vi "HFRR ADV v036.vi"() -> ()   [LabVIEW 2025] (continued)
            n1884 = local write "Main Dashboard Buttons"(T1."Advance" ("Main Dashboard Buttons")) -> ()
          }
        }
      }
    }
    n1885 = case shown="True" "Prog Uno" {
      frame False {
      }
      frame True {
        n1886 = stacked-sequence {
          frame #0 {
            n1887 = Delete(path (use dialog)=path "C:/LAB-IQ-NXT/UNOCOMPILE.bat" ("working directory")) -> ()  [unwired: 4 in, 3 out]
          }
          frame #1 {
            n1888 = local read "Com Port 1"() -> (w2646:refnum<visa-resource-name>)
            n1889 = Concatenate Strings("cmd.exe /c \"mode " ("command line"), w2646, ":1200,n,8,1\"\n" ("command line")) -> (w2651:string)
            n1890 = Concatenate Strings(w2651, "CD\\\nCD WinDucom\navrdude -C avrdude.conf -v -patmega328p -carduino -P" ("command line"), w2646, " -b115200 -D -Uflash:w:UNO_V20.hex:i\n" ("command line"), "\r") -> (w2653:string)
            "STR" <- w2653
            n1891 = call <vilib>:"Write Characters To File.vi"("append to file? (new file:F)"=FALSE, "character string"=w2653, "file path (dialog if empty)"=path "C:/LAB-IQ/UNOCOMPILE.bat" ("working directory")) -> ()  [unwired: 2 in, 1 out]
          }
          frame #2 {
            n1892 = disable-structure shown="Disabled" {
              frame Disabled {
                w2657 = "cmd.exe  /c \"C:\\LAB-IQ-NXT\\UNOCOMPILE.bat\"" ("string")
                n1893 = local write "Prog Uno"(FALSE ("run minimized? (F)")) -> ()
                n1894 = call <vilib>:"System Exec.vi"("expected output size  (4096)"=u32 65535, "run minimized? (F)"=FALSE, "wait until completion? (T)"=TRUE ("run minimized? (F)"), "working directory"=path "C:/LAB-IQ-NXT", "standard input"=w2657, "command line"=w2657) -> ("error out"=w2656:errorcluster, "standard output"=→"String 42":string)  [unwired: 2 in, 2 out]
                "error out 3" <- w2656
                n1895 = flat-sequence {
                  tunnel: w2656 -> [_]
                  frame #0 {
                  }
                }
              }
              frame Enabled {
              }
            }
          }
        }
      }
    }
    n1896 = case shown="\"ISO 12156\"" "TEST STANDARD" {
      frame "ASTM D6079", Default {
        w2626 = 50.0 ("Hz")
        w2627 = 53.0 ("Set Rh")
        w2629 = 1.0 ("Set Strk")
        w2628 = 60.0 ("Set Temp")
        # "astm hide"
        n1897 = local write "NORMAL LOAD"(200.0 ("NORMAL LOAD")) -> ()
        n1898 = local write "Set Strk"(w2629) -> ()
        n1899 = local write "Set Hz"(w2626) -> ()
        n1900 = local write "Set Temp"(w2628) -> ()
        n1901 = local write "Set Rh"(w2627) -> ()
        n1902 = local write "test time"(75.0 ("test time")) -> ()
        n1903 = local write "Set Stroke:"(w2629) -> ()
        n1904 = local write "Set Humidity:"(w2627) -> ()
        n1905 = local write "Set Frequency:"(w2626) -> ()
        n1906 = local write "Set Temperature:"(w2628) -> ()
        "Test Standard" <- "ASTM D6079" ("Test Standard 2")
      }
      frame "ISO 12156" {
        n1907 = local write "Set Strk"(1.0 ("Set Strk")) -> ()
        n1908 = local write "NORMAL LOAD"(200.0 ("NORMAL LOAD")) -> ()
        n1909 = local write "Set Temp"(60.0 ("Set Temp")) -> ()
        n1910 = local write "test time"(75.0 ("test time")) -> ()
        n1911 = local write "Set Hz"(50.0 ("Hz")) -> ()
        n1912 = local write "Set Rh"(53.0 ("Set Rh")) -> ()
      }
      frame "CEC F-096-A-06" {
        n1913 = local write "Set Strk"(1.0 ("Set Strk")) -> ()
        n1914 = local write "NORMAL LOAD"(200.0 ("NORMAL LOAD")) -> ()
        n1915 = local write "Set Temp"(60.0 ("Set Temp")) -> ()
        n1916 = local write "test time"(75.0 ("test time")) -> ()
        n1917 = local write "Set Hz"(50.0 ("Hz")) -> ()
        n1918 = local write "Set Rh"(53.0 ("Set Rh")) -> ()
      }
      frame "Custom" {
      }
    }
    n1919 = Or(x=w2179, y=w2177) -> (x .or. y?=w2178:bool)
    n1920 = case shown="\"About\"" w2176 {
      tunnel: [T29."Acquire" ("Main Tab") T29."Compare Files" ("Main Tab") T29."About" ("Main Tab")] -> w2187
      frame "Acquire", Default {
      }
      frame "Compare Files" {
      }
      frame "About" {
      }
    }
    n1921 = Or(x=w2182, y="OPEN") -> (x .or. y?=w2183:bool)
    n1922 = case shown="True" w2183 {
      tunnel: w2182 -> [_ w2215]
      frame False {
      }
      frame True {
        n1923 = stacked-sequence {
          tunnel: w2215 -> [_ w2282 _ _]
          frame #0 {
            w2231 = "  " ("String 6")
            n1924 = local write "OPEN"(FALSE ("open")) -> ()
            n1925 = local read "string1 2"() -> (w2219:string)
            n1926 = local read "string1 3"() -> (w2218:string)
            n1927 = local read "string1 4"() -> (w2217:string)
            n1928 = property on="OPEN" class="Bool (strict)"("Visible"=FALSE) -> ()  [unwired: 2 in, 2 out]
            n1929 = local write "String 6"(w2231) -> ()
            n1930 = local write "String 7"(w2231) -> ()
            n1931 = local write "String 8"(w2231) -> ()
            n1932 = local write "String 12"(w2231) -> ()
            n1933 = local read "OK Button 16"() -> (w2216:bool)
            n1934 = String To Path(string=w2219) -> (path=w2227:path)
            n1935 = String To Path(string=w2218) -> (path=w2226:path)
            n1936 = String To Path(string=w2217) -> (path=w2225:path)
            n1937 = case shown="True" w2216 {
              tunnel: [w2232 w2233] -> w2220
              frame False {
                n1938 = local read "string1"() -> (w2232:string)
              }
              frame True {
                n1939 = local read "String Indicator 4"() -> (w2233:string)
              }
            }
            n1940 = Open/Create/Replace File "Open File"(file path (use dialog)=w2227) -> (refnum out=w2223:refnum<file>)  [unwired: 5 in, 2 out]
            n1941 = Open/Create/Replace File "Open File"(file path (use dialog)=w2226) -> (refnum out=w2222:refnum<file>)  [unwired: 5 in, 2 out]
            n1942 = Open/Create/Replace File "Open File"(file path (use dialog)=w2225) -> (refnum out=w2221:refnum<file>)  [unwired: 5 in, 2 out]
            n1943 = while {
              tunnel: w2223 -> [w2245]
              i -> [w2241]
              stop <- w2240 continue-if-true
              (unwired) TRUE ("line mode (F)")
              n1944 = Read from Text File "Read File"(file (use dialog)=w2245) -> (text=w2242:string)  [unwired: 3 in, 3 out]
              n1945 = local write "Numeric 11"(w2241) -> ()
              n1946 = String Length(string=w2242) -> (length=w2244:i32)
              n1947 = Greater?(x=w2244, y=1) -> (0:w2240:bool)
            }
            n1948 = while {
              tunnel: w2222 -> [w2251]
              i -> [w2247]
              stop <- w2246 continue-if-true
              (unwired) TRUE ("line mode (F)")
              n1949 = Read from Text File "Read File"(file (use dialog)=w2251) -> (text=w2248:string)  [unwired: 3 in, 3 out]
              n1950 = local write "Numeric 12"(w2247) -> ()
              n1951 = String Length(string=w2248) -> (length=w2250:i32)
              n1952 = Greater?(x=w2250, y=1) -> (0:w2246:bool)
            }
            n1953 = while {
              tunnel: w2221 -> [w2257]
              i -> [w2253]
              stop <- w2252 continue-if-true
              (unwired) TRUE ("line mode (F)")
              n1954 = Read from Text File "Read File"(file (use dialog)=w2257) -> (text=w2254:string)  [unwired: 3 in, 3 out]
              n1955 = local write "Numeric 13"(w2253) -> ()
              n1956 = String Length(string=w2254) -> (length=w2256:i32)
              n1957 = Greater?(x=w2256, y=1) -> (0:w2252:bool)
            }
            n1958 = String To Path(string=w2220) -> (path=w2228:path)
            n1959 = Open/Create/Replace File "Open File"(file path (use dialog)=w2228) -> (refnum out=w2224:refnum<file>)  [unwired: 5 in, 2 out]
            n1960 = while {
              tunnel: w2224 -> [w2239]
              i -> [w2235]
              stop <- w2234 continue-if-true
              (unwired) TRUE ("line mode (F)")
              n1961 = Read from Text File "Read File"(file (use dialog)=w2239) -> (text=w2236:string)  [unwired: 3 in, 3 out]
              n1962 = local write "Numeric 8"(w2235) -> ()
              n1963 = String Length(string=w2236) -> (length=w2238:i32)
              n1964 = Greater?(x=w2238, y=1) -> (0:w2234:bool)
            }
          }
          frame #1 {
            w2409 = FALSE ("ACTUAL   MERGE")
            # "Sample Temp"
            # "ECR"
            # "COF"
            # "Time\nCOF\nFF\nTemp"
            n1965 = case shown="True" w2282 {
              tunnel: [w2429 w2430] -> w2283
              frame False {
                n1966 = local read "string1"() -> (w2429:string)
              }
              frame True {
                n1967 = local read "String Indicator 4"() -> (w2430:string)
              }
            }
            n1968 = local read "string1 3"() -> (w2327:string)
            n1969 = String To Path(string=w2283) -> (path=w2414:path)
            n1970 = String To Path(string=w2327) -> (path=w2425:path)
            n1971 = local read "Numeric 12"() -> (w2411:i32)
            n1972 = local read "Numeric 8"() -> (w2413:i32)
            n1973 = local read "string1 2"() -> (w2328:string)
            n1974 = local read "string1 4"() -> (w2326:string)
            n1975 = Open/Create/Replace File "Open File"(file path (use dialog)=w2414) -> (refnum out=w2428:refnum<file>, error out=w2427:errorcluster)  [unwired: 5 in, 1 out]
            n1976 = Open/Create/Replace File "Open File"(file path (use dialog)=w2425) -> (refnum out=w2421:refnum<file>, error out=w2422:errorcluster)  [unwired: 5 in, 1 out]
            n1977 = for {
              N: w2413 -> [_]
              tunnel: w2428 -> [w2576]
              tunnel: w2427 -> [w2575]
              tunnel: [w2565] -> w2340 mode=indexing
              tunnel: [w2563] -> w2397 mode=indexing
              tunnel: [w2564] -> w2392 mode=indexing
              tunnel: w2409 -> [_]
              tunnel: [w2557] -> w2394 mode=indexing
              tunnel: [w2553] -> w2363 mode=indexing
              tunnel: [w2549] -> w2338 mode=indexing
              tunnel: [w2545] -> w2319 mode=indexing
              tunnel: [w2540] -> w2279 mode=indexing
              (unwired) TRUE ("line mode (F)")
              # "freq"
              # "Stroke"
              # "Time"
              # "CoF"
              # "Humidity"
              # "Temp"
              # "Air Temp"
              # "ECR"
              n1978 = Read from Text File "Read File"(file (use dialog)=w2576, error in=w2575) -> (text=w2541:string)  [unwired: 2 in, 3 out]
              n1979 = local write "String 6"(w2541) -> ()
              n1980 = String Subset(string=w2541, offset (0)=0, length (rest)=14 ("length (rest)")) -> (substring=w2569:string)
              n1981 = String Subset(string=w2541, offset (0)=35, length (rest)=9 ("length (rest)")) -> (substring=w2566:string)
              n1982 = String Subset(string=w2541, offset (0)=15, length (rest)=9 ("length (rest)")) -> (substring=w2572:string)
              n1983 = Fract/Exp String To Number(string=w2569) -> (number=w2565:dbl)  [unwired: 3 in, 1 out]
              n1984 = Fract/Exp String To Number(string=w2566) -> (number=w2564:dbl)  [unwired: 3 in, 1 out]
              n1985 = Fract/Exp String To Number(string=w2572) -> (number=w2563:dbl)  [unwired: 3 in, 1 out]
              n1986 = String Subset(string=w2541, offset (0)=85, length (rest)=9 ("length (rest)")) -> (substring=w2542:string)
              n1987 = String Subset(string=w2541, offset (0)=25, length (rest)=9 ("length (rest)")) -> (substring=w2548:string)
              n1988 = String Subset(string=w2541, offset (0)=55, length (rest)=9 ("length (rest)")) -> (substring=w2550:string)
              n1989 = String Subset(string=w2541, offset (0)=45, length (rest)=9 ("length (rest)")) -> (substring=w2556:string)
              n1990 = String Subset(string=w2541, offset (0)=65, length (rest)=9 ("length (rest)")) -> (substring=w2562:string)
              n1991 = Fract/Exp String To Number(string=w2548) -> (number=w2545:dbl)  [unwired: 3 in, 1 out]
              n1992 = Fract/Exp String To Number(string=w2542) -> (number=w2540:dbl)  [unwired: 3 in, 1 out]
              n1993 = Fract/Exp String To Number(string=w2550) -> (number=w2549:dbl)  [unwired: 3 in, 1 out]
              n1994 = Fract/Exp String To Number(string=w2556) -> (number=w2553:dbl)  [unwired: 3 in, 1 out]
              n1995 = Fract/Exp String To Number(string=w2562) -> (number=w2559:dbl)  [unwired: 3 in, 1 out]
              n1996 = Add(x=w2559, y=0.0) -> (x+y=w2557:dbl)
            }
            n1997 = for {
              N: w2411 -> [_]
              tunnel: w2422 -> [w2502]
              tunnel: w2421 -> [w2501]
              tunnel: [w2491] -> w2380 mode=indexing
              tunnel: [w2489] -> w2378 mode=indexing
              tunnel: [w2490] -> w2374 mode=indexing
              tunnel: w2409 -> [_]
              tunnel: [w2483] -> w2376 mode=indexing
              tunnel: [w2479] -> w2358 mode=indexing
              tunnel: [w2475] -> w2334 mode=indexing
              tunnel: [w2472] -> w2315 mode=indexing
              tunnel: [w2468] -> w2274 mode=indexing
              (unwired) 9 ("length (rest)")
              (unwired) 9 ("length (rest)")
              (unwired) TRUE ("line mode (F)")
              n1998 = Read from Text File "Read File"(file (use dialog)=w2501, error in=w2502) -> (text=w2469:string)  [unwired: 2 in, 3 out]
              n1999 = local write "String 8"(w2469) -> ()
              n2000 = String Subset(string=w2469, offset (0)=85) -> (substring=w2471:string)  [unwired: 1 in]
              n2001 = String Subset(string=w2469, offset (0)=35, length (rest)=9 ("length (rest)")) -> (substring=w2492:string)
              n2002 = String Subset(string=w2469, offset (0)=55, length (rest)=9 ("length (rest)")) -> (substring=w2477:string)
              n2003 = String Subset(string=w2469, offset (0)=25) -> (substring=w2473:string)  [unwired: 1 in]
              n2004 = String Subset(string=w2469, offset (0)=15, length (rest)=9 ("length (rest)")) -> (substring=w2498:string)
              n2005 = String Subset(string=w2469, offset (0)=0, length (rest)=14 ("length (rest)")) -> (substring=w2495:string)
              n2006 = String Subset(string=w2469, offset (0)=45, length (rest)=9 ("length (rest)")) -> (substring=w2482:string)
              n2007 = String Subset(string=w2469, offset (0)=65, length (rest)=9 ("length (rest)")) -> (substring=w2488:string)
              n2008 = Fract/Exp String To Number(string=w2471) -> (number=w2468:dbl)  [unwired: 3 in, 1 out]
              n2009 = Fract/Exp String To Number(string=w2492) -> (number=w2490:dbl)  [unwired: 3 in, 1 out]
              n2010 = Fract/Exp String To Number(string=w2477) -> (number=w2475:dbl)  [unwired: 3 in, 1 out]
              n2011 = Fract/Exp String To Number(string=w2473) -> (number=w2472:dbl)  [unwired: 3 in, 1 out]
              n2012 = Fract/Exp String To Number(string=w2498) -> (number=w2489:dbl)  [unwired: 3 in, 1 out]
              n2013 = Fract/Exp String To Number(string=w2495) -> (number=w2491:dbl)  [unwired: 3 in, 1 out]
              n2014 = Fract/Exp String To Number(string=w2482) -> (number=w2479:dbl)  [unwired: 3 in, 1 out]
              n2015 = Fract/Exp String To Number(string=w2488) -> (number=w2485:dbl)  [unwired: 3 in, 1 out]
              n2016 = Add(x=w2485, y=0.0) -> (x+y=w2483:dbl)
            }
            n2017 = String To Path(string=w2328) -> (path=w2426:path)
            n2018 = String To Path(string=w2326) -> (path=w2420:path)
            n2019 = local read "Numeric 11"() -> (w2410:i32)
            n2020 = local read "Numeric 13"() -> (w2412:i32)
            n2021 = Open/Create/Replace File "Open File"(file path (use dialog)=w2426) -> (refnum out=w2424:refnum<file>, error out=w2423:errorcluster)  [unwired: 5 in, 1 out]
            n2022 = Open/Create/Replace File "Open File"(file path (use dialog)=w2420) -> (refnum out=w2419:refnum<file>, error out=w2418:errorcluster)  [unwired: 5 in, 1 out]
            n2023 = for {
              N: w2410 -> [_]
              tunnel: w2424 -> [w2539]
              tunnel: w2423 -> [w2538]
              tunnel: [w2528] -> w2390 mode=indexing
              tunnel: [w2526] -> w2388 mode=indexing
              tunnel: [w2527] -> w2383 mode=indexing
              tunnel: w2409 -> [_]
              tunnel: [w2520] -> w2385 mode=indexing
              tunnel: [w2516] -> w2361 mode=indexing
              tunnel: [w2512] -> w2336 mode=indexing
              tunnel: [w2508] -> w2317 mode=indexing
              tunnel: [w2503] -> w2275 mode=indexing
              (unwired) TRUE ("line mode (F)")
              n2024 = Read from Text File "Read File"(file (use dialog)=w2539, error in=w2538) -> (text=w2504:string)  [unwired: 2 in, 3 out]
              n2025 = local write "String 7"(w2504) -> ()
              n2026 = String Subset(string=w2504, offset (0)=85, length (rest)=9 ("length (rest)")) -> (substring=w2507:string)
              n2027 = String Subset(string=w2504, offset (0)=35, length (rest)=9 ("length (rest)")) -> (substring=w2529:string)
              n2028 = String Subset(string=w2504, offset (0)=55, length (rest)=9 ("length (rest)")) -> (substring=w2515:string)
              n2029 = String Subset(string=w2504, offset (0)=25, length (rest)=9 ("length (rest)")) -> (substring=w2509:string)
              n2030 = String Subset(string=w2504, offset (0)=45, length (rest)=9 ("length (rest)")) -> (substring=w2517:string)
              n2031 = String Subset(string=w2504, offset (0)=0, length (rest)=14 ("length (rest)")) -> (substring=w2532:string)
              n2032 = String Subset(string=w2504, offset (0)=15, length (rest)=9 ("length (rest)")) -> (substring=w2535:string)
              n2033 = String Subset(string=w2504, offset (0)=65, length (rest)=9 ("length (rest)")) -> (substring=w2521:string)
              n2034 = Fract/Exp String To Number(string=w2507) -> (number=w2503:dbl)  [unwired: 3 in, 1 out]
              n2035 = Fract/Exp String To Number(string=w2529) -> (number=w2527:dbl)  [unwired: 3 in, 1 out]
              n2036 = Fract/Exp String To Number(string=w2515) -> (number=w2512:dbl)  [unwired: 3 in, 1 out]
              n2037 = Fract/Exp String To Number(string=w2509) -> (number=w2508:dbl)  [unwired: 3 in, 1 out]
              n2038 = Fract/Exp String To Number(string=w2517) -> (number=w2516:dbl)  [unwired: 3 in, 1 out]
              n2039 = Fract/Exp String To Number(string=w2532) -> (number=w2528:dbl)  [unwired: 3 in, 1 out]
              n2040 = Fract/Exp String To Number(string=w2535) -> (number=w2526:dbl)  [unwired: 3 in, 1 out]
              n2041 = Fract/Exp String To Number(string=w2521) -> (number=w2524:dbl)  [unwired: 3 in, 1 out]
              n2042 = Add(x=w2524, y=0.0) -> (x+y=w2520:dbl)
            }
            n2043 = for {
              N: w2412 -> [_]
              tunnel: w2419 -> [w2467]
              tunnel: w2418 -> [w2466]
              tunnel: [w2456] -> w2372 mode=indexing
              tunnel: [w2455] -> w2365 mode=indexing
              tunnel: w2409 -> [_]
              tunnel: [w2444] -> w2370 mode=indexing
              tunnel: [w2449] -> w2367 mode=indexing
              tunnel: [w2445] -> w2357 mode=indexing
              tunnel: [w2440] -> w2332 mode=indexing
              tunnel: [w2436] -> w2313 mode=indexing
              tunnel: [w2431] -> w2273 mode=indexing
              (unwired) 1.0 ("x")
              (unwired) TRUE ("line mode (F)")
              n2044 = Read from Text File "Read File"(file (use dialog)=w2467, error in=w2466) -> (text=w2432:string)  [unwired: 2 in, 3 out]
              n2045 = local write "String 12"(w2432) -> ()
              n2046 = String Subset(string=w2432, offset (0)=85, length (rest)=9 ("length (rest)")) -> (substring=w2434:string)
              n2047 = String Subset(string=w2432, offset (0)=35, length (rest)=9 ("length (rest)")) -> (substring=w2457:string)
              n2048 = String Subset(string=w2432, offset (0)=55, length (rest)=9 ("length (rest)")) -> (substring=w2442:string)
              n2049 = String Subset(string=w2432, offset (0)=25, length (rest)=9 ("length (rest)")) -> (substring=w2438:string)
              n2050 = String Subset(string=w2432, offset (0)=45, length (rest)=9 ("length (rest)")) -> (substring=w2447:string)
              n2051 = String Subset(string=w2432, offset (0)=15, length (rest)=9 ("length (rest)")) -> (substring=w2463:string)
              n2052 = String Subset(string=w2432, offset (0)=0, length (rest)=14 ("length (rest)")) -> (substring=w2460:string)
              n2053 = String Subset(string=w2432, offset (0)=65, length (rest)=9 ("length (rest)")) -> (substring=w2450:string)
              n2054 = Fract/Exp String To Number(string=w2434) -> (number=w2431:dbl)  [unwired: 3 in, 1 out]
              n2055 = Fract/Exp String To Number(string=w2457) -> (number=w2455:dbl)  [unwired: 3 in, 1 out]
              n2056 = Fract/Exp String To Number(string=w2442) -> (number=w2440:dbl)  [unwired: 3 in, 1 out]
              n2057 = Fract/Exp String To Number(string=w2438) -> (number=w2436:dbl)  [unwired: 3 in, 1 out]
              n2058 = Fract/Exp String To Number(string=w2447) -> (number=w2445:dbl)  [unwired: 3 in, 1 out]
              n2059 = Fract/Exp String To Number(string=w2463) -> (number=w2444:dbl)  [unwired: 3 in, 1 out]
              n2060 = Fract/Exp String To Number(string=w2460) -> (number=w2456:dbl)  [unwired: 3 in, 1 out]
              n2061 = Fract/Exp String To Number(string=w2450) -> (number=w2453:dbl)  [unwired: 3 in, 1 out]
              n2062 = Add(x=w2453, y=0.0) -> (x+y=w2449:dbl)
            }
            n2063 = Delete From Array(array=w2315, index=0) -> (array with subset deleted=w2288:dbl[])  [unwired: 1 in, 1 out]
            n2064 = Delete From Array(array=w2378, index=0) -> (array with subset deleted=w2351:dbl[])  [unwired: 1 in, 1 out]
            n2065 = Delete From Array(array=w2358, index=0) -> (array with subset deleted=w2346:dbl[])  [unwired: 1 in, 1 out]
            n2066 = Delete From Array(array=w2376, index=0) -> (array with subset deleted=w2377:dbl[])  [unwired: 1 in, 1 out]
            n2067 = call-poly <vilib>:"Mean.vi"("X"=w2288) -> ("mean"=→"КОФ2 4":dbl)  [unwired: 1 out]
            n2068 = call-poly <vilib>:"Mean.vi"("X"=w2351) -> ("mean"=→"КОФ3":dbl)  [unwired: 1 out]
            n2069 = call-poly <vilib>:"Mean.vi"("X"=w2346) -> ("mean"=→"CP3":dbl)  [unwired: 1 out]
            n2070 = Delete From Array(array=w2340, index=0) -> (array with subset deleted=w2267:dbl[])  [unwired: 1 in, 1 out]
            n2071 = Delete From Array(array=w2279, index=0) -> (array with subset deleted=w2266:dbl[])  [unwired: 1 in, 1 out]
            n2072 = Delete From Array(array=w2319, index=0) -> (array with subset deleted=w2290:dbl[])  [unwired: 1 in, 1 out]
            n2073 = Delete From Array(array=w2397, index=0) -> (array with subset deleted=w2352:dbl[])  [unwired: 1 in, 1 out]
            n2074 = Delete From Array(array=w2363, index=0) -> (array with subset deleted=w2348:dbl[])  [unwired: 1 in, 1 out]
            "array w/ subset deleted" <- w2348
            n2075 = Delete From Array(array=w2394, index=0) -> (array with subset deleted=w2395:dbl[])  [unwired: 1 in, 1 out]
            n2076 = call-poly <vilib>:"Mean.vi"("X"=w2290) -> ("mean"=→"КОФ2 2":dbl)  [unwired: 1 out]
            n2077 = call-poly <vilib>:"Mean.vi"("X"=w2352) -> ("mean"=→"КОФ1":dbl)  [unwired: 1 out]
            n2078 = Bundle "Bundle"(w2267, w2266) -> (w2272:cluster{dbl[], dbl[]})  [unwired: 1 in]
            n2079 = Bundle "Bundle"(w2267, w2395) -> (w2259:cluster{dbl[], dbl[]})  [unwired: 1 in]
            n2080 = Delete From Array(array=w2274, index=0) -> (array with subset deleted=w2262:dbl[])  [unwired: 1 in, 1 out]
            n2081 = Delete From Array(array=w2275, index=0) -> (array with subset deleted=w2264:dbl[])  [unwired: 1 in, 1 out]
            n2082 = Delete From Array(array=w2385, index=0) -> (array with subset deleted=w2386:dbl[])  [unwired: 1 in, 1 out]
            n2083 = Delete From Array(array=w2273, index=0) -> (array with subset deleted=w2260:dbl[])  [unwired: 1 in, 1 out]
            n2084 = Delete From Array(array=w2367, index=0) -> (array with subset deleted=w2368:dbl[])  [unwired: 1 in, 1 out]
            n2085 = Delete From Array(array=w2392, index=0) -> (array with subset deleted=w2298:dbl[])  [unwired: 1 in, 1 out]
            n2086 = Delete From Array(array=w2338, index=0) -> (array with subset deleted=w2294:dbl[])  [unwired: 1 in, 1 out]
            n2087 = Delete From Array(array=w2374, index=0) -> (array with subset deleted=w2296:dbl[])  [unwired: 1 in, 1 out]
            n2088 = Delete From Array(array=w2334, index=0) -> (array with subset deleted=w2292:dbl[])  [unwired: 1 in, 1 out]
            n2089 = Delete From Array(array=w2383, index=0) -> (array with subset deleted=w2297:dbl[])  [unwired: 1 in, 1 out]
            n2090 = Delete From Array(array=w2336, index=0) -> (array with subset deleted=w2293:dbl[])  [unwired: 1 in, 1 out]
            n2091 = Delete From Array(array=w2317, index=0) -> (array with subset deleted=w2289:dbl[])  [unwired: 1 in, 1 out]
            n2092 = Delete From Array(array=w2361, index=0) -> (array with subset deleted=w2347:dbl[])  [unwired: 1 in, 1 out]
            n2093 = Delete From Array(array=w2388, index=0) -> (array with subset deleted=w2349:dbl[])  [unwired: 1 in, 1 out]
            n2094 = Delete From Array(array=w2365, index=0) -> (array with subset deleted=w2295:dbl[])  [unwired: 1 in, 1 out]
            n2095 = Delete From Array(array=w2332, index=0) -> (array with subset deleted=w2291:dbl[])  [unwired: 1 in, 1 out]
            n2096 = Delete From Array(array=w2313, index=0) -> (array with subset deleted=w2287:dbl[])  [unwired: 1 in, 1 out]
            n2097 = Delete From Array(array=w2357, index=0) -> (array with subset deleted=w2345:dbl[])  [unwired: 1 in, 1 out]
            n2098 = Delete From Array(array=w2370, index=0) -> (array with subset deleted=w2350:dbl[])  [unwired: 1 in, 1 out]
            n2099 = Delete From Array(array=w2380, index=0) -> (array with subset deleted=w2263:dbl[])  [unwired: 1 in, 1 out]
            n2100 = Delete From Array(array=w2390, index=0) -> (array with subset deleted=w2265:dbl[])  [unwired: 1 in, 1 out]
            n2101 = Delete From Array(array=w2372, index=0) -> (array with subset deleted=w2261:dbl[])  [unwired: 1 in, 1 out]
            n2102 = Bundle "Bundle"(w2267, w2298) -> (w2285:cluster{dbl[], dbl[]})  [unwired: 1 in]
            n2103 = Bundle "Bundle"(w2267, w2352) -> (w2286:cluster{dbl[], dbl[]})  [unwired: 1 in]
            n2104 = Bundle "Bundle"(w2298, w2294) -> (w2300:cluster{dbl[], dbl[]})  [unwired: 1 in]
            n2105 = Bundle "Bundle"(w2263, w2262) -> (w2270:cluster{dbl[], dbl[]})  [unwired: 1 in]
            n2106 = Bundle "Bundle"(w2296, w2292) -> (w2302:cluster{dbl[], dbl[]})  [unwired: 1 in]
            n2107 = Bundle "Bundle"(w2263, w2296) -> (w2406:cluster{dbl[], dbl[]})  [unwired: 1 in]
            n2108 = Bundle "Bundle"(w2263, w2292) -> (w2330:cluster{dbl[], dbl[]})  [unwired: 1 in]
            n2109 = Bundle "Bundle"(w2263, w2351) -> (w2416:cluster{dbl[], dbl[]})  [unwired: 1 in]
            n2110 = Bundle "Bundle"(w2263, w2346) -> (w2354:cluster{dbl[], dbl[]})  [unwired: 1 in]
            n2111 = Bundle "Bundle"(w2263, w2377) -> (w2401:cluster{dbl[], dbl[]})  [unwired: 1 in]
            n2112 = Bundle "Bundle"(w2297, w2293) -> (w2301:cluster{dbl[], dbl[]})  [unwired: 1 in]
            n2113 = Bundle "Bundle"(w2265, w2264) -> (w2271:cluster{dbl[], dbl[]})  [unwired: 1 in]
            n2114 = Bundle "Bundle"(w2265, w2297) -> (w2408:cluster{dbl[], dbl[]})  [unwired: 1 in]
            n2115 = Bundle "Bundle"(w2265, w2293) -> (w2331:cluster{dbl[], dbl[]})  [unwired: 1 in]
            n2116 = Bundle "Bundle"(w2265, w2347) -> (w2355:cluster{dbl[], dbl[]})  [unwired: 1 in]
            n2117 = Bundle "Bundle"(w2265, w2349) -> (w2417:cluster{dbl[], dbl[]})  [unwired: 1 in]
            n2118 = Bundle "Bundle"(w2265, w2386) -> (w2399:cluster{dbl[], dbl[]})  [unwired: 1 in]
            n2119 = Bundle "Bundle"(w2295, w2291) -> (w2303:cluster{dbl[], dbl[]})  [unwired: 1 in]
            n2120 = Bundle "Bundle"(w2261, w2260) -> (w2269:cluster{dbl[], dbl[]})  [unwired: 1 in]
            n2121 = Bundle "Bundle"(w2261, w2295) -> (w2407:cluster{dbl[], dbl[]})  [unwired: 1 in]
            n2122 = Bundle "Bundle"(w2261, w2291) -> (w2329:cluster{dbl[], dbl[]})  [unwired: 1 in]
            n2123 = Bundle "Bundle"(w2261, w2345) -> (w2353:cluster{dbl[], dbl[]})  [unwired: 1 in]
            n2124 = Bundle "Bundle"(w2261, w2350) -> (w2415:cluster{dbl[], dbl[]})  [unwired: 1 in]
            n2125 = Bundle "Bundle"(w2261, w2368) -> (w2400:cluster{dbl[], dbl[]})  [unwired: 1 in]
            n2126 = call-poly <vilib>:"Mean.vi"("X"=w2348) -> ("mean"=→"CP1":dbl)  [unwired: 1 out]
            n2127 = call-poly <vilib>:"Mean.vi"("X"=w2289) -> ("mean"=→"КОФ2 3":dbl)  [unwired: 1 out]
            n2128 = call-poly <vilib>:"Mean.vi"("X"=w2347) -> ("mean"=→"CP2":dbl)  [unwired: 1 out]
            n2129 = call-poly <vilib>:"Mean.vi"("X"=w2349) -> ("mean"=→"КОФ2":dbl)  [unwired: 1 out]
            n2130 = call-poly <vilib>:"Mean.vi"("X"=w2287) -> ("mean"=→"КОФ2 5":dbl)  [unwired: 1 out]
            n2131 = call-poly <vilib>:"Mean.vi"("X"=w2345) -> ("mean"=→"CP4":dbl)  [unwired: 1 out]
            n2132 = call-poly <vilib>:"Mean.vi"("X"=w2350) -> ("mean"=→"КОФ4":dbl)  [unwired: 1 out]
            n2133 = Bundle "Bundle"(w2267, w2294) -> (w2258:cluster{dbl[], dbl[]})  [unwired: 1 in]
            n2134 = Bundle "Bundle"(w2267, w2348) -> (w2281:cluster{dbl[], dbl[]})  [unwired: 1 in]
            n2135 = Build Array "Build Array"(w2258, w2281) -> (w2284:cluster{dbl[], dbl[]}[])
            "XY Graph 17" <- w2284
            n2136 = Build Array "Build Array"(w2272, w2271, w2270, w2269) -> (→"Frequency ( Hz )":cluster{dbl[], dbl[]}[])
            n2137 = Build Array "Build Array"(w2300, w2301, w2302, w2303) -> (→"Air Temp ( °C ) vs Humidity ( % RH )":cluster{dbl[], dbl[]}[])
            n2138 = Build Array "Build Array"(w2285, w2408, w2406, w2407) -> (→"Air Temperature  ( °C )":cluster{dbl[], dbl[]}[])
            n2139 = Build Array "Build Array"(w2258, w2331, w2330, w2329) -> (→"Humidity ( %RH )":cluster{dbl[], dbl[]}[])
            n2140 = Build Array "Build Array"(w2286, w2417, w2416, w2415) -> (→"Coefficient Of Friction":cluster{dbl[], dbl[]}[])
            n2141 = Build Array "Build Array"(w2281, w2355, w2354, w2353) -> (→"Sample Temperature ( °C )":cluster{dbl[], dbl[]}[])
            n2142 = Build Array "Build Array"(w2259, w2399, w2401, w2400) -> (→"XY Graph 13":cluster{dbl[], dbl[]}[])
            n2143 = Bundle "Bundle"(w2267, w2290) -> (w2312:cluster{dbl[], dbl[]})  [unwired: 1 in]
            n2144 = Bundle "Bundle"(w2263, w2288) -> (w2310:cluster{dbl[], dbl[]})  [unwired: 1 in]
            n2145 = Bundle "Bundle"(w2265, w2289) -> (w2311:cluster{dbl[], dbl[]})  [unwired: 1 in]
            n2146 = Bundle "Bundle"(w2261, w2287) -> (w2309:cluster{dbl[], dbl[]})  [unwired: 1 in]
            n2147 = Build Array "Build Array"(w2312, w2311, w2310, w2309) -> (→"Stroke ( mm )":cluster{dbl[], dbl[]}[])
            n2148 = local write "XY Graph 16"(w2284) -> ()
          }
          frame #2 {
          }
          frame #3 {
            n2149 = local write "Numeric 8"(0 ("Numeric 8")) -> ()
            n2150 = local write "Numeric 11"(0 ("Numeric 11")) -> ()
            n2151 = local write "Numeric 12"(0 ("Numeric 12")) -> ()
            n2152 = local write "Numeric 13"(0 ("Numeric 13")) -> ()
            n2153 = property on="OPEN" class="Bool (strict)"("Visible"=TRUE) -> ()  [unwired: 2 in, 2 out]
            n2154 = local read "String Control 2"() -> (w2584:string)
            n2155 = local read "String Control 4"() -> (w2583:string)
            n2156 = local read "String Control 6"() -> (w2582:string)
            n2157 = local read "String Control 8"() -> (w2581:string)
            n2158 = Match Pattern(string=w2584, regular expression="Samples / cycle :- ") -> (after substring=w2598:string)  [unwired: 1 in, 3 out]
            n2159 = Match Pattern(string=w2584, regular expression="Frequency :- ") -> (after substring=w2617:string)  [unwired: 1 in, 3 out]
            n2160 = Match Pattern(string=w2583, regular expression="Samples / cycle :- ") -> (after substring=w2594:string)  [unwired: 1 in, 3 out]
            n2161 = Match Pattern(string=w2583, regular expression="Frequency :- ") -> (after substring=w2612:string)  [unwired: 1 in, 3 out]
            n2162 = Match Pattern(string=w2582, regular expression="Samples / cycle :- ") -> (after substring=w2590:string)  [unwired: 1 in, 3 out]
            n2163 = Match Pattern(string=w2582, regular expression="Frequency :- ") -> (after substring=w2607:string)  [unwired: 1 in, 3 out]
            n2164 = Match Pattern(string=w2581, regular expression="Samples / cycle :- ") -> (after substring=w2586:string)  [unwired: 1 in, 3 out]
            n2165 = Match Pattern(string=w2581, regular expression="Frequency :- ") -> (after substring=w2602:string)  [unwired: 1 in, 3 out]
            n2166 = String Subset(string=w2598, length (rest)=6 ("length (rest)")) -> (substring=w2600:string)  [unwired: 1 in]
            n2167 = String Subset(string=w2617, length (rest)=9 ("length (rest)")) -> (substring=w2619:string)  [unwired: 1 in]
            n2168 = String Subset(string=w2594, length (rest)=6 ("length (rest)")) -> (substring=w2596:string)  [unwired: 1 in]
            n2169 = String Subset(string=w2612, length (rest)=9 ("length (rest)")) -> (substring=w2614:string)  [unwired: 1 in]
            n2170 = String Subset(string=w2590, length (rest)=6 ("length (rest)")) -> (substring=w2592:string)  [unwired: 1 in]
            n2171 = String Subset(string=w2607, length (rest)=9 ("length (rest)")) -> (substring=w2609:string)  [unwired: 1 in]
            n2172 = String Subset(string=w2586, length (rest)=6 ("length (rest)")) -> (substring=w2588:string)  [unwired: 1 in]
            n2173 = String Subset(string=w2602, length (rest)=9 ("length (rest)")) -> (substring=w2604:string)  [unwired: 1 in]
            n2174 = Fract/Exp String To Number(string=w2600) -> (number=w2580:dbl)  [unwired: 3 in, 1 out]
            n2175 = Fract/Exp String To Number(string=w2619) -> (number=w2620:dbl)  [unwired: 3 in, 1 out]
            n2176 = Fract/Exp String To Number(string=w2596) -> (number=w2579:dbl)  [unwired: 3 in, 1 out]
            n2177 = Fract/Exp String To Number(string=w2614) -> (number=w2615:dbl)  [unwired: 3 in, 1 out]
            n2178 = Fract/Exp String To Number(string=w2592) -> (number=w2578:dbl)  [unwired: 3 in, 1 out]
            n2179 = Fract/Exp String To Number(string=w2609) -> (number=w2610:dbl)  [unwired: 3 in, 1 out]
            n2180 = Fract/Exp String To Number(string=w2588) -> (number=w2577:dbl)  [unwired: 3 in, 1 out]
            n2181 = Fract/Exp String To Number(string=w2604) -> (number=w2605:dbl)  [unwired: 3 in, 1 out]
            n2182 = local write "sample1"(w2580) -> ()
            n2183 = local write "freq1"(w2620) -> ()
            n2184 = local write "sample2"(w2579) -> ()
            n2185 = local write "freq2"(w2615) -> ()
            n2186 = local write "sample3"(w2578) -> ()
            n2187 = local write "freq3"(w2610) -> ()
            n2188 = local write "sample4"(w2577) -> ()
            n2189 = local write "freq 4"(w2605) -> ()
          }
        }
      }
    }
    n2190 = case shown="True" w2178 {
      selector: w2178 -> [_ w2197]
      frame False {
      }
      frame True {
        n2191 = Not(x=w2197) -> (.not. x?=w2193:bool)
        n2192 = local write "service 3"(w2193) -> ()
        n2193 = local write "OPEN 6"(w2193) -> ()
        n2194 = call <vilib>:"System Exec.vi"("wait until completion? (T)"=TRUE, "command line"="C:\\LAB-IQ\\Scar View.exe") -> ("error out"=→"error out 5":errorcluster)  [unwired: 6 in, 3 out]
      }
    }
    n2195 = case shown="\"Acquire\", Default" w2187 {
      frame "Acquire", Default {
        # "Elapsed time\ncof\nstroke\nAir temp\nTemp\nHumidity"
        n2196 = disable-structure shown="Disabled" {
          frame Disabled {
            n2197 = local read "Flag"() -> (w2896:dbl)
            n2198 = local read "RUN"() -> (w2893:bool)
            n2199 = Not(x=w2893) -> (.not. x?=w2892:bool)
            n2200 = Equal?(x=w2896, y=10.0) -> (x = y?=w2894:bool)
            n2201 = And(x=w2894, y=w2892) -> (x .and. y?=w2891:bool)
            n2202 = case shown="True" w2891 {
              frame False {
              }
              frame True {
                w2897 = FALSE ("Heater Button")
                n2203 = local write "Humidity"(w2897) -> ()
                n2204 = local write "Heater Button"(w2897) -> ()
              }
            }
          }
          frame Enabled {
          }
        }
        n2205 = disable-structure shown="Disabled" {
          frame Disabled {
            n2206 = case shown="True" {
              selector: _ -> [_ _]
              frame False {
              }
              frame True {
                w2942 = TRUE ("Heater")
                n2207 = local write "Humidity"(w2942) -> ()
                n2208 = local write "Heater Button"(w2942) -> ()
                n2209 = local read "TEST STANDARD"() -> (w2945:T3)
                n2210 = local read "TEST STANDARD"() -> (w2940:T3)
                n2211 = Equal?(x=w2945, y=enum16{"ASTM D6079", "ISO 12156", "Custom"}."ISO 12156" ("Test Standard")) -> (x = y?=w2943:bool)
                n2212 = Equal?(x=w2940, y=enum16{"ASTM D6079", "ISO 12156", "Custom"}."ASTM D6079" ("Test Standard")) -> (x = y?=w2939:bool)
                n2213 = case shown="True" w2943 {
                  frame False {
                  }
                  frame True {
                    n2214 = local write "airtempflg"(FALSE ("airtempflg")) -> ()
                    n2215 = local write item#-1(TRUE ("Heater")) -> ()
                  }
                }
                n2216 = case shown="True" w2939 {
                  frame False {
                  }
                  frame True {
                    n2217 = local write "airtempflg"(TRUE ("airtempflg")) -> ()
                    n2218 = local write item#-1(FALSE ("Heater")) -> ()
                  }
                }
              }
            }
          }
          frame Enabled {
          }
        }
        n2219 = stacked-sequence {
          frame #0 {
            n2220 = case shown="True" "RST FF" {
              frame False {
              }
              frame True {
                w2959 = 0.0 ("X Scale.Range:Maximum")
                n2221 = property on="Frictional Force ( N )" class="WFChart (strict)"("XScale.Maximum"=600.0 ("X Scale.Range:Maximum"), "XScale.Minimum"=w2959, "YScale.Maximum"=10.0 ("Y Scale.Range:Maximum"), "YScale.Minimum"=w2959) -> ()  [unwired: 2 in, 2 out]
              }
            }
          }
          frame #1 {
            n2222 = case shown="True" "RST TEMP" {
              frame False {
              }
              frame True {
                n2223 = property on="Temperature ( Deg C )" class="WFChart (strict)"("XScale.Minimum"=0.0 ("X Scale.Range:Minimum"), "XScale.Maximum"=600.0 ("X Scale.Range:Maximum"), "YScale.Minimum"=0.0 ("Y Scale.Range:Minimum"), "YScale.Maximum"=100.0 ("Y Scale.Range:Maximum")) -> ()  [unwired: 2 in, 2 out]
              }
            }
          }
          frame #2 {
            n2224 = case shown="True" "RSTCOF" {
              frame False {
              }
              frame True {
                n2225 = property on="Coefficient of Friction" class="WFChart (strict)"("XScale.Minimum"=0.0 ("X Scale.Range:Minimum"), "XScale.Maximum"=600.0 ("X Scale.Range:Maximum"), "YScale.Maximum"=1.0 ("X Scale.Range:Minimum"), "YScale.Minimum"=0.0 ("X Scale.Range:Minimum")) -> ()  [unwired: 2 in, 2 out]
              }
            }
          }
          frame #3 {
            n2226 = case shown="True" "RSTCOF 2" {
              frame False {
              }
              frame True {
                (unwired) 100.0 ("Y Scale.Range:Maximum")
                (unwired) 0.0 ("Y Scale.Range:Minimum")
                (unwired) 600.0 ("X Scale.Range:Maximum")
                (unwired) 0.0 ("X Scale.Range:Minimum")
              }
            }
          }
          frame #4 {
            n2227 = case shown="True" "RSTCOF 3" {
              frame False {
              }
              frame True {
                n2228 = property on="Electrical Contact Resistance ( % )" class="WFChart (strict)"("XScale.Minimum"=0.0 ("X Scale.Range:Minimum"), "XScale.Maximum"=600.0 ("X Scale.Range:Maximum"), "YScale.Minimum"=0.0 ("Y Scale.Range:Minimum"), "YScale.Maximum"=100.0 ("Y Scale.Range:Maximum")) -> ()  [unwired: 2 in, 2 out]
              }
            }
          }
        }
        n2229 = local read "RUN"() -> (w2886:bool)
        n2230 = case shown="False" w2886 {
          frame False {
          }
          frame True {
          }
        }
        n2231 = local read "RUN"() -> (w2890:bool)
        n2232 = case shown="False" w2890 {
          tunnel: [FALSE ("TEST RUNNING") TRUE ("TEST RUNNING")] -> w2889
          frame False {
            w2978 = 0.0 ("Flag")
            n2233 = local write "Elapsed time"(0.0 ("elapsedtime")) -> ()
            n2234 = local write "Time Remaining"(w2978) -> ()
            n2235 = local write "Flag"(w2978) -> ()
            n2236 = local write "Remaining Time"(w2978) -> ()
          }
          frame True {
            n2237 = local write "Flag"(10.0 ("Flag")) -> ()
          }
        }
        n2238 = local read "AIR TEMP"() -> (w2884:dbl)
        n2239 = Greater Or Equal?(x=w2884, y=15.0) -> (x >= y?=w2885:bool)
        "powstat" <- w2885
        n2240 = case shown="True" "Save & Continue" {
          frame False {
          }
          frame True {
            n2241 = local read "USER ID"() -> (w3280:string)
            n2242 = local read "FILE"() -> (w3288:string)
            n2243 = String Length(string=w3288) -> (length=w3286:i32)
            n2244 = String Length(string=w3280) -> (length=w3283:i32)
            n2245 = Greater?(x=w3286, y=0) -> (0:w3285:bool)
            n2246 = Greater?(x=w3283, y=0) -> (0:w3282:bool)
            n2247 = And(x=w3285, y=w3282) -> (x .and. y?=w3281:bool)
            n2248 = case shown="True" w3281 {
              frame False {
                n2249 = stacked-sequence {
                  frame #0 {
                    n2250 = One Button Dialog(message="Please Enter a File Name and Operator ID to save data !", button name ("OK")="Ok") -> ()  [unwired: 1 out]
                  }
                  frame #1 {
                    n2251 = local write "Save & Continue"(FALSE ("OK Button")) -> ()
                  }
                }
                n2252 = local write "Save & Continue"(FALSE ("OK Button")) -> ()
              }
              frame True {
                n2253 = stacked-sequence {
                  frame #0 {
                    n2254 = local read "FILE"() -> (w3294:string)
                    n2255 = call "file check.vi"("file name in"=w3294) -> ("file name out"=w3293:string)  [unwired: 9 in, 1 out]
                    n2256 = call <vilib>:"Application Directory.vi"() -> ("Application Directory"=w3304:path)
                    n2257 = Build Path(base path=w3304, name or relative path="data") -> (appended path=w3303:path)
                    n2258 = call <vilib>:"Trim Whitespace.vi"("string"=w3293) -> ("trimmed string"=w3301:string)  [unwired: 1 in]
                    n2259 = call <vilib>:"Trim Whitespace.vi"("string"=w3293) -> ("trimmed string"=w3302:string)  [unwired: 1 in]
                    n2260 = List Folder(path=w3303) -> (folder names=w3299:string[])  [unwired: 3 in, 3 out]
                    n2261 = Match Pattern(string=w3301, regular expression="_(") -> (before substring=w3298:string)  [unwired: 1 in, 3 out]
                    n2262 = for {
                      tunnel: w3299 -> [w3313] mode=indexing
                      tunnel: w3298 -> [w3311]
                      shift-right: [w3309] -> w3296
                      shift-left: bool[] [] -> [w3310]
                      n2263 = Match Pattern(string=w3313, regular expression="_(") -> (before substring=w3312:string)  [unwired: 1 in, 3 out]
                      n2264 = Equal?(x=w3312, y=w3311) -> (x = y?=w3308:bool)
                      n2265 = case shown="True" w3308 {
                        tunnel: w3308 -> [_ w3316]
                        tunnel: w3310 -> [w3315 w3318]
                        tunnel: [w3315 w3317] -> w3309
                        frame False {
                        }
                        frame True {
                          n2266 = Insert Into Array(array=w3318, new element=w3316) -> (w3317:bool[])  [unwired: 1 in]
                        }
                      }
                    }
                    n2267 = Equal?(x=w3299, y=w3298) -> (x = y?=w3307:bool[])
                    n2268 = Or Array Elements(Boolean array=w3307) -> (logical OR=w3306:bool)
                    n2269 = Array Size(array=w3296) -> (size(s)=w3295:i32)
                    n2270 = case shown="True" w3306 {
                      tunnel: w3302 -> [_ w3326]
                      tunnel: w3295 -> [_ w3319]
                      frame False {
                      }
                      frame True {
                        n2271 = Number To Decimal String(number=w3319) -> (decimal integer string=w3322:string)  [unwired: 1 in]
                        n2272 = Search/Split String(string=w3326, search string/char (-)="_(" ("regular expression")) -> (substring before match=w3324:string)  [unwired: 1 in, 2 out]
                        n2273 = Concatenate Strings(w3324, "_(" ("regular expression"), w3322, ")" ("regular expression")) -> (w3320:string)
                        n2274 = local write "FILE"(w3320) -> ()
                      }
                    }
                  }
                  frame #1 {
                    w3329 = 0.0
                    w3342 = cluster{"y":dbl, dbl, "y":dbl}[] [] ("History Data")
                    w3343 = FALSE ("Heater Button")
                    (unwired) ")!" ("string")
                    (unwired) ")" ("string")
                    w3341 = dbl[] [] ("History Data")
                    w3347 = "\r"
                    # "C:\\WinDucom\\Data\\"
                    # "C:\\LAB-IQ-NXT\\data"
                    n2275 = local write "Humidity ( %RH )"(w3329) -> ()
                    n2276 = local write "Frequency ( Hz )"(w3329) -> ()
                    n2277 = local write "Stroke 3"(w3329) -> ()
                    n2278 = local write "speedop"(0.0 ("PIDclk 2")) -> ()
                    n2279 = local write "Set Temp 2"(65.0 ("Set Temp 2")) -> ()
                    n2280 = local write "AIR TEMP"(w3329) -> ()
                    n2281 = local write "clk"(0.0 ("clk")) -> ()
                    n2282 = local write "Stroke 4"(w3329) -> ()
                    n2283 = local write "COF 2"(w3329) -> ()
                    n2284 = local write "TEMP"(w3329) -> ()
                    n2285 = local write "ecr 3"(w3329) -> ()
                    n2286 = local write "FF 3"(w3329) -> ()
                    n2287 = local write "FF 2"(w3329) -> ()
                    n2288 = property on="Coefficient of Friction" class="WFChart (strict)"("History Data"=w3341) -> ()  [unwired: 2 in, 2 out]
                    n2289 = property on="Coefficient of Friction" class="WFChart (strict)"("History Data"=w3341) -> ()  [unwired: 2 in, 2 out]
                    n2290 = property on="Frictional Force ( N )" class="WFChart (strict)"("History Data"=w3341) -> ()  [unwired: 2 in, 2 out]
                    n2291 = property on="Electrical Contact Resistance ( % )" class="WFChart (strict)"("History Data"=w3341) -> ()  [unwired: 2 in, 2 out]
                    n2292 = property on="Electrical Contact Resistance ( % )" class="WFChart (strict)"("History Data"=w3341) -> ()  [unwired: 2 in, 2 out]
                    n2293 = property on="Temperature ( Deg C )" class="WFChart (strict)"("History Data"=w3341) -> ()  [unwired: 2 in, 2 out]
                    n2294 = property on="Frictional Force ( N )" class="WFChart (strict)"("History Data"=w3341) -> ()  [unwired: 2 in, 2 out]
                    n2295 = property on="Coefficient of Friction" class="WFChart (strict)"("History Data"=w3341) -> ()  [unwired: 2 in, 2 out]
                    n2296 = property on="Frictional Force ( N )" class="WFChart (strict)"("History Data"=w3341) -> ()  [unwired: 2 in, 2 out]
                    n2297 = property on="Electrical Contact Resistance ( % )" class="WFChart (strict)"("History Data"=w3341) -> ()  [unwired: 2 in, 2 out]
                    n2298 = property on="Temperature ( Deg C )" class="WFChart (strict)"("History Data"=w3341) -> ()  [unwired: 2 in, 2 out]
                    n2299 = property on="Stroke ( mm )" class="WFChart (strict)"("History Data"=w3342) -> ()  [unwired: 2 in, 2 out]
                    n2300 = property on="Stroke ( mm )" class="WFChart (strict)"("History Data"=w3342) -> ()  [unwired: 2 in, 2 out]
                    n2301 = local write "Humidity"(w3343) -> ()
                    n2302 = local write "Heater Button"(w3343) -> ()
                    n2303 = local read "FILE"() -> (w3337:string)
                    n2304 = disable-structure shown="Enabled" {
                      disable-tunnel: [w3381 _] -> w3328
                      frame Enabled {
                        n2305 = local read "NORMAL LOAD"() -> (w3381:dbl)
                      }
                      frame Disabled {
                      }
                    }
                    n2306 = call "file check.vi"("file name in"=w3337) -> ("error out"=w3340:errorcluster, "file name out"=w3334:string)  [unwired: 9 in]
                    n2307 = call "FILE PATH CREATION.vi"("error in"=w3340, "FILE NAME :"=w3334) -> ("FILE OUT"=w3333:path)  [unwired: 8 in, 1 out]
                    n2308 = Concatenate Strings(w3334, ".dgf" ("Substring")) -> (w3339:string)
                    n2309 = Concatenate Strings(w3334, ".duf" ("Substring")) -> (w3335:string)
                    n2310 = Multiply(x=w3328, y=1.0) -> (x*y=w3360:dbl)
                    n2311 = Build Path(base path=w3333, name or relative path=w3339) -> (appended path=w3332:path)
                    n2312 = Build Path(base path=w3333, name or relative path=w3335) -> (appended path=w3331:path)
                    n2313 = Number To Fractional String(number=w3360, width (-)=i16 5, precision (6)=i16 2) -> (F-format string=w3368:string)  [unwired: 1 in]
                    n2314 = local read "tested by"() -> (w3327:string)
                    n2315 = local read "Fuel Discription :"() -> (w3356:string)
                    n2316 = local read "Batch Ref Num :"() -> (w3345:string)
                    n2317 = Get Date/Time String(date format (0)=enum16{"short", "long", "abbreviated"}."short") -> (date string=w3379:string, time string=w3376:string)  [unwired: 2 in]
                    n2318 = local read "Remarks :"() -> (w3355:string)
                    n2319 = Concatenate Strings("Load :- " ("Substring"), w3368, " grams ," ("Substring")) -> (w3367:string)
                    n2320 = local read "String 41"() -> (w3348:string)
                    n2321 = Concatenate Strings(w3356) -> (w3357:string)
                    n2322 = Concatenate Strings(w3345) -> (w3344:string)
                    n2323 = Concatenate Strings(w3327) -> (w3351:string)
                    n2324 = Concatenate Strings("(" ("Substring"), w3379, ")" ("Substring"), w3376) -> (w3350:string)
                    "concatenated string" <- w3350
                    n2325 = Concatenate Strings(w3355, "," ("string")) -> (w3354:string)
                    n2326 = Concatenate Strings("  TIME;      COF;       STROKE;     AIR TEMP;  TEMP;  HUMIDITY;  ECR; PID-OUT; FREQUENCY" ("Substring"), "\r") -> (w3363:string)
                    n2327 = Concatenate Strings(w3348, w3347, "Fuel Discription :-" ("Substring"), w3357, w3347, w3367, w3347, "Batch Ref Num :-" ("Substring"), w3344, w3347, " Remarks :- " ("Substring"), w3354, w3347, " Date :- " ("Substring"), w3350, w3347, "Tested By :-" ("Substring"), w3351) -> (w3361:string)
                    "REMARKS" <- w3361
                    n2328 = call <vilib>:"Write Characters To File.vi"("append to file? (new file:F)"=FALSE, "character string"=w3363, "file path (dialog if empty)"=w3332) -> ()  [unwired: 2 in, 1 out]
                    n2329 = call <vilib>:"Write Characters To File.vi"("append to file? (new file:F)"=FALSE, "character string"=w3361, "file path (dialog if empty)"=w3331) -> ()  [unwired: 2 in, 1 out]
                  }
                  frame #2 {
                    n2330 = local write "Cycles elapsed"(0 ("Cycles elapsed")) -> ()
                    n2331 = local write "cyclecount"(0 ("cyclecount")) -> ()
                    n2332 = local write "Save & Continue"(FALSE ("OK")) -> ()
                    n2333 = local write "autostrtflg"(TRUE ("autostrtflg")) -> ()
                    n2334 = local write "Save"(FALSE ("Save")) -> ()
                    n2335 = Get Date/Time In Seconds() -> (seconds since 1Jan1904=w3386:timestamp)
                    n2336 = To Double Precision Float(number=w3386) -> (double precision float=w3385:dbl)
                    n2337 = local write "acq timer"(w3385) -> ()
                    n2338 = One Button Dialog(message="Please ensure sample is mounted properly and machine is ready in all aspects for testing !", button name ("OK")="Ok") -> ()  [unwired: 1 out]
                  }
                  frame #3 {
                    n2339 = stacked-sequence {
                      frame #0 {
                        n2340 = local write "Main Dashboard Buttons"(T1."Dashboard" ("Main Dashboard Buttons")) -> ()
                        n2341 = local write "Main Tab"(T2."Acquire" ("Main Tab")) -> ()
                      }
                      frame #1 {
                        n2342 = local write "EVENT LOG"("" ("EVENT LOG")) -> ()
                      }
                      frame #2 {
                        n2343 = Wait (ms)(milliseconds to wait=u32 50) -> ()  [unwired: 1 out]
                      }
                      frame #3 {
                        n2344 = disable-structure shown="Disabled" {
                          frame Disabled {
                            n2345 = local read "EVENT LOG"() -> (w3398:string)
                            n2346 = call "Event Log.vi"("Content"="Test Details", "EVENT LOG"=w3398) -> ("EVENT LOG"=w3397:string)  [unwired: 8 in, 1 out]
                            n2347 = local write "EVENT LOG"(w3397) -> ()
                          }
                          frame Enabled {
                          }
                        }
                      }
                      frame #4 {
                        n2348 = Wait (ms)(milliseconds to wait=u32 50) -> ()  [unwired: 1 out]
                      }
                      frame #5 {
                        n2349 = local read "FILE"() -> (w3400:string)
                        n2350 = Concatenate Strings("File Name :" ("Content"), w3400) -> (w3401:string)
                        n2351 = local read "EVENT LOG"() -> (w3404:string)
                        n2352 = call "Event Log.vi"("Content"=w3401, "EVENT LOG"=w3404) -> ("EVENT LOG"=w3403:string)  [unwired: 8 in, 1 out]
                        n2353 = local write "EVENT LOG"(w3403) -> ()
                      }
                      frame #6 {
                        n2354 = Wait (ms)(milliseconds to wait=u32 50) -> ()  [unwired: 1 out]
                      }
                      frame #7 {
                        n2355 = local read "Batch Ref Num :"() -> (w3406:string)
                        n2356 = Concatenate Strings("Batch Ref No :" ("Content"), w3406) -> (w3407:string)
                        n2357 = local read "EVENT LOG"() -> (w3410:string)
                        n2358 = call "Event Log.vi"("Content"=w3407, "EVENT LOG"=w3410) -> ("EVENT LOG"=w3409:string)  [unwired: 8 in, 1 out]
                        n2359 = local write "EVENT LOG"(w3409) -> ()
                      }
                      frame #8 {
                        n2360 = Wait (ms)(milliseconds to wait=u32 50) -> ()  [unwired: 1 out]
                      }
                      frame #9 {
                        n2361 = local read "tested by"() -> (w3412:string)
                        n2362 = Concatenate Strings("Tested By :" ("Content"), w3412) -> (w3413:string)
                        n2363 = local read "EVENT LOG"() -> (w3416:string)
                        n2364 = call "Event Log.vi"("Content"=w3413, "EVENT LOG"=w3416) -> ("EVENT LOG"=w3415:string)  [unwired: 8 in, 1 out]
                        n2365 = local write "EVENT LOG"(w3415) -> ()
                      }
                      frame #10 {
                        n2366 = Wait (ms)(milliseconds to wait=u32 50) -> ()  [unwired: 1 out]
                      }
                      frame #11 {
                        n2367 = local read "TEST STANDARD"() -> (w3419:T3)
                        n2368 = case shown="\"ASTM D6079\", Default" w3419 {
                          tunnel: ["ASTM D6079" "ISO 12156" "CEC F-096-A-06" "Custom"] -> w3418
                          frame "ASTM D6079", Default {
                          }
                          frame "ISO 12156" {
                          }
                          frame "CEC F-096-A-06" {
                          }
                          frame "Custom" {
                          }
                        }
                        n2369 = Concatenate Strings("Test Standard :" ("Content"), w3418) -> (w3420:string)
                        n2370 = local read "EVENT LOG"() -> (w3423:string)
                        n2371 = call "Event Log.vi"("Content"=w3420, "EVENT LOG"=w3423) -> ("EVENT LOG"=w3422:string)  [unwired: 8 in, 1 out]
                        n2372 = local write "EVENT LOG"(w3422) -> ()
                      }
                      frame #12 {
                        n2373 = Wait (ms)(milliseconds to wait=u32 50) -> ()  [unwired: 1 out]
                      }
                      frame #13 {
                        n2374 = local read "Fuel Discription :"() -> (w3429:string)
                        n2375 = Concatenate Strings("Fuel Description :" ("Content"), w3429) -> (w3430:string)
                        n2376 = local read "EVENT LOG"() -> (w3433:string)
                        n2377 = call "Event Log.vi"("Content"=w3430, "EVENT LOG"=w3433) -> ("EVENT LOG"=w3432:string)  [unwired: 8 in, 1 out]
                        n2378 = local write "EVENT LOG"(w3432) -> ()
                      }
                      frame #14 {
                        n2379 = Wait (ms)(milliseconds to wait=u32 50) -> ()  [unwired: 1 out]
                      }
                      frame #15 {
                        n2380 = local read "Remarks :"() -> (w3435:string)
                        n2381 = Concatenate Strings("Remarks :" ("Content"), w3435) -> (w3436:string)
                        n2382 = local read "EVENT LOG"() -> (w3439:string)
                        n2383 = call "Event Log.vi"("Content"=w3436, "EVENT LOG"=w3439) -> ("EVENT LOG"=w3438:string)  [unwired: 8 in, 1 out]
                        n2384 = local write "EVENT LOG"(w3438) -> ()
                      }
                      frame #16 {
                        n2385 = Wait (ms)(milliseconds to wait=u32 50) -> ()  [unwired: 1 out]
                      }
                      frame #17 {
                        n2386 = local read "USER ID"() -> (w3441:string)
                        n2387 = Concatenate Strings("Operator ID :" ("Content"), w3441) -> (w3443:string)
                        n2388 = local read "EVENT LOG"() -> (w3445:string)
                        n2389 = call "Event Log.vi"("Content"=w3443, "EVENT LOG"=w3445) -> ("EVENT LOG"=w3444:string)  [unwired: 8 in, 1 out]
                        n2390 = local write "EVENT LOG"(w3444) -> ()
                      }
                      frame #18 {
                        n2391 = Wait (ms)(milliseconds to wait=u32 50) -> ()  [unwired: 1 out]
                      }
                      frame #19 {
                        n2392 = disable-structure shown="Disabled" {
                          frame Disabled {
                            n2393 = local read "EVENT LOG"() -> (w3449:string)
                            n2394 = call "Event Log.vi"("Content"="Test Parameter", "EVENT LOG"=w3449) -> ("EVENT LOG"=w3448:string)  [unwired: 8 in, 1 out]
                            n2395 = local write "EVENT LOG"(w3448) -> ()
                          }
                          frame Enabled {
                          }
                        }
                      }
                      frame #20 {
                        n2396 = Wait (ms)(milliseconds to wait=u32 50) -> ()  [unwired: 1 out]
                      }
                      frame #21 {
                        n2397 = local read "Set Hz"() -> (w3453:dbl)
                        n2398 = Number To Fractional String(number=w3453, precision (6)=i16 2) -> (F-format string=w3452:string)  [unwired: 2 in]
                        n2399 = Concatenate Strings("Set Frequency [Hz] :" ("Content"), w3452) -> (w3455:string)
                        n2400 = local read "EVENT LOG"() -> (w3457:string)
                        n2401 = call "Event Log.vi"("Content"=w3455, "EVENT LOG"=w3457) -> ("EVENT LOG"=w3456:string)  [unwired: 8 in, 1 out]
                        n2402 = local write "EVENT LOG"(w3456) -> ()
                      }
                      frame #22 {
                        n2403 = Wait (ms)(milliseconds to wait=u32 50) -> ()  [unwired: 1 out]
                      }
                      frame #23 {
